vi "Update Splash Screen.vi"(8 "error in (no error)":errorcluster, 10 "Close Splash Screen?":bool, 11 "Splash Screen Status":string) -> (0 "error out":errorcluster)   [LabVIEW 2016, in "SLL Splash Screen.lvlib"]
doc: "API for updating the status text in the splash screen and to control when the splash screen has to be closed."
uses:
  SLL Splash Screen.lvlib
  _Typedefs/Splash Screen Data.ctl
  _Typedefs/User Event LV2 Command.ctl
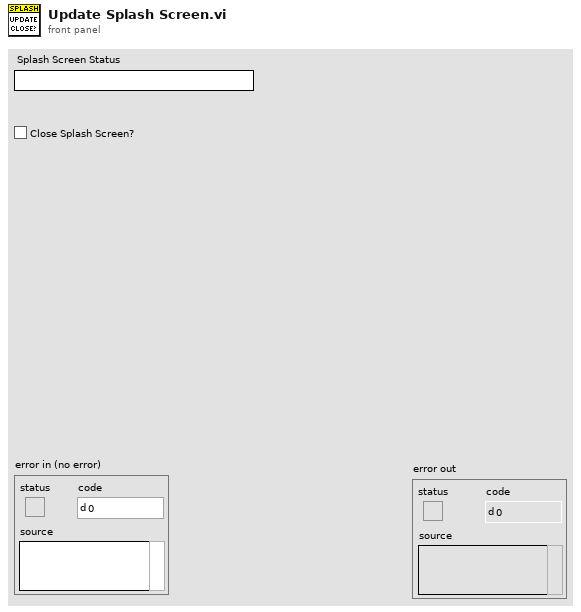
[diagram p1: front panel]
types:
  T1 = typedef "SLL Splash Screen.lvlib/User Event LV2 Command.ctl" = enum16{"Create", "Generate", "Delete"}
  T2 = typedef "SLL Splash Screen.lvlib/Splash Screen Data.ctl" = cluster{"Status":string, "Close?":bool}
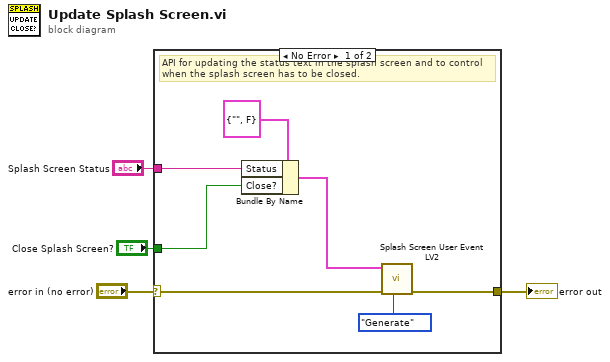
[diagram p0: block diagram]
diagram:
  n1 = case shown="No Error" "error in (no error)" {
    selector: "error in (no error)" -> [w8 w12]
    tunnel: [w7 w12] -> w3
    tunnel: "Splash Screen Status" -> [w10 _]
    tunnel: "Close Splash Screen?" -> [w9 _]
    frame No Error {
      # "API for updating the status text in the splash screen and to control when the splash screen has to be closed."
      n2 = Bundle By Name(cluster=T2 {"Status"="", "Close?"=FALSE} ("Splash Screen"), "Status"=w10, "Close?"=w9) -> (w6:T2)
      n3 = call "Splash Screen User Event LV2.vi"("Command"=User_Event_LV2_Command."Generate", "error in (no error)"=w8, "Splash Screen"=w6) -> ("error out"=w7:errorcluster)  [unwired: 7 in, 1 out]
    }
    frame Error {
    }
  }
  "error out" <- w3
